vi "VI UUT.vi"(9 "Boolean Control":bool, 10 "String Control":string, 11 "Numeric Control":dbl) -> (1 "Boolean Indicator":bool, 2 "String Indicator":string, 3 "Numeric Indicator":dbl)   [LabVIEW 2020, in "Test Scripting API.lvclass"]
uses:
  Test Scripting API.lvclass
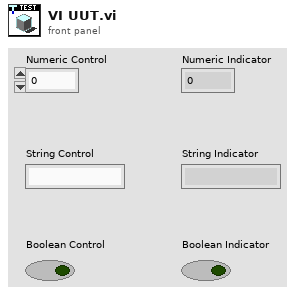
[diagram p1: front panel]
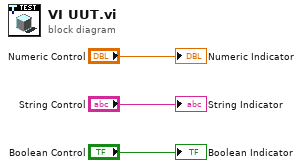
[diagram p0: block diagram]
diagram:
  "Numeric Indicator" <- "Numeric Control"
  "String Indicator" <- "String Control"
  "Boolean Indicator" <- "Boolean Control"
